vi "oef16.vi"() -> ()   [LabVIEW 2021]
panel:
  in  "upper-case":bool
  out "output":string
  in  "input":string
  # "lower-case"
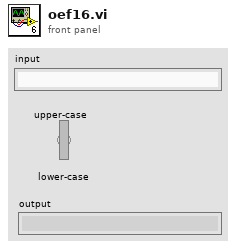
[diagram p1: front panel]
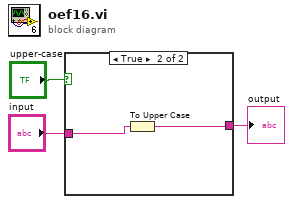
[diagram p0: block diagram]
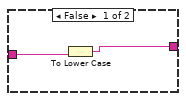
[diagram p2: hidden frame]
diagram:
  n1 = case shown="True" "upper-case" {
    tunnel: "input" -> [w5 w7]
    tunnel: [w4 w6] -> w1
    frame False {
      n2 = To Lower Case(string=w5) -> (all lower case string=w4:string)
    }
    frame True {
      n3 = To Upper Case(1:w7) -> (0:w6:string)
    }
  }
  "output" <- w1
